vi "PAN_SetGlobalPaths.vi"(6 "macro in":path, 7 "common in":path, 9 "modules in":path, 10 "logs in":path, 11 "configs in":path) -> ()   [LabVIEW 2016]
uses:
  Modules/DBSHAND/private/vis/DatabaseHand_Element_Set(path).vi
  Modules/DBSHAND/private/vis/DatabaseHand_Element_Set(string).vi
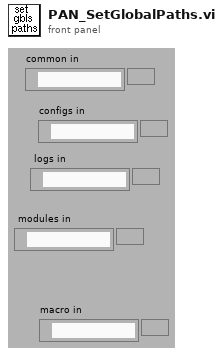
[diagram p1: front panel]
types:
  T1 = typedef "DatabaseHand_RefNum.ctl" = refnum<vi>
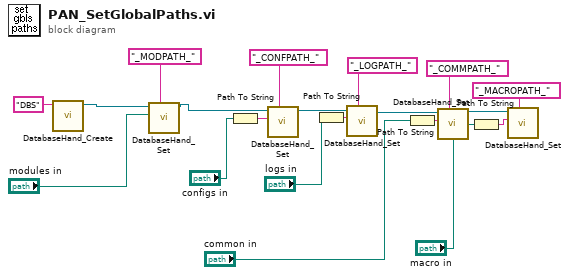
[diagram p0: block diagram]
diagram:
  n1 = call "DatabaseHand_Create.vi"("Name"="DBS") -> ("Database RefNum out"=w19:T1)  [unwired: 1 in, 9 out]
  n2 = call-poly "DatabaseHand_Set.vi"("name"="_MODPATH_" ("group"), "value"="modules in", "Database RefNum in"=w19) -> ("Database RefNum out"=w17:T1)  [unwired: 5 in, 3 out]
  n3 = Path To String(path="configs in") -> (string=w11:string)
  n4 = call-poly "DatabaseHand_Set.vi"("name"="_CONFPATH_" ("group"), "value"=w11, "Database RefNum in"=w17) -> ("Database RefNum out"=w14:T1)  [unwired: 5 in, 3 out]
  n5 = Path To String(path="logs in") -> (string=w10:string)
  n6 = call-poly "DatabaseHand_Set.vi"("name"="_LOGPATH_" ("group"), "value"=w10, "Database RefNum in"=w14) -> ("Database RefNum out"=w6:T1)  [unwired: 5 in, 3 out]
  n7 = Path To String(path="common in") -> (string=w7:string)
  n8 = call-poly "DatabaseHand_Set.vi"("name"="_COMMPATH_" ("group"), "value"=w7, "Database RefNum in"=w6) -> ("Database RefNum out"=w4:T1)  [unwired: 5 in, 3 out]
  n9 = Path To String(path="macro in") -> (string=w2:string)
  n10 = call-poly "DatabaseHand_Set.vi"("name"="_MACROPATH_", "value"=w2, "Database RefNum in"=w4) -> ()  [unwired: 5 in, 4 out]
